vi "areaModify.vi"(3 "区域信息":T1 {"电极排列方式" items=["等间隔十字排列", "等间隔一字排列", "等间隔错误排列"]}, 8 "error in (no error)":errorcluster caption="错误输入（无错误）", 11 "编号":dbl) -> (0 "error out (no error) 2":errorcluster caption="错误输出（无错误）", 1 "连接的字符串":string)   [LabVIEW 2014, in "SettingD.lvlib"]
uses:
  SettingD.llb/SettingD.lvlib
  DataBase/DataBase.lvlib
panel:
  out "area_id":string
  out "结果字符串":string
  in  "取消按钮":bool
  in  "确定按钮":bool
  out "元素":string
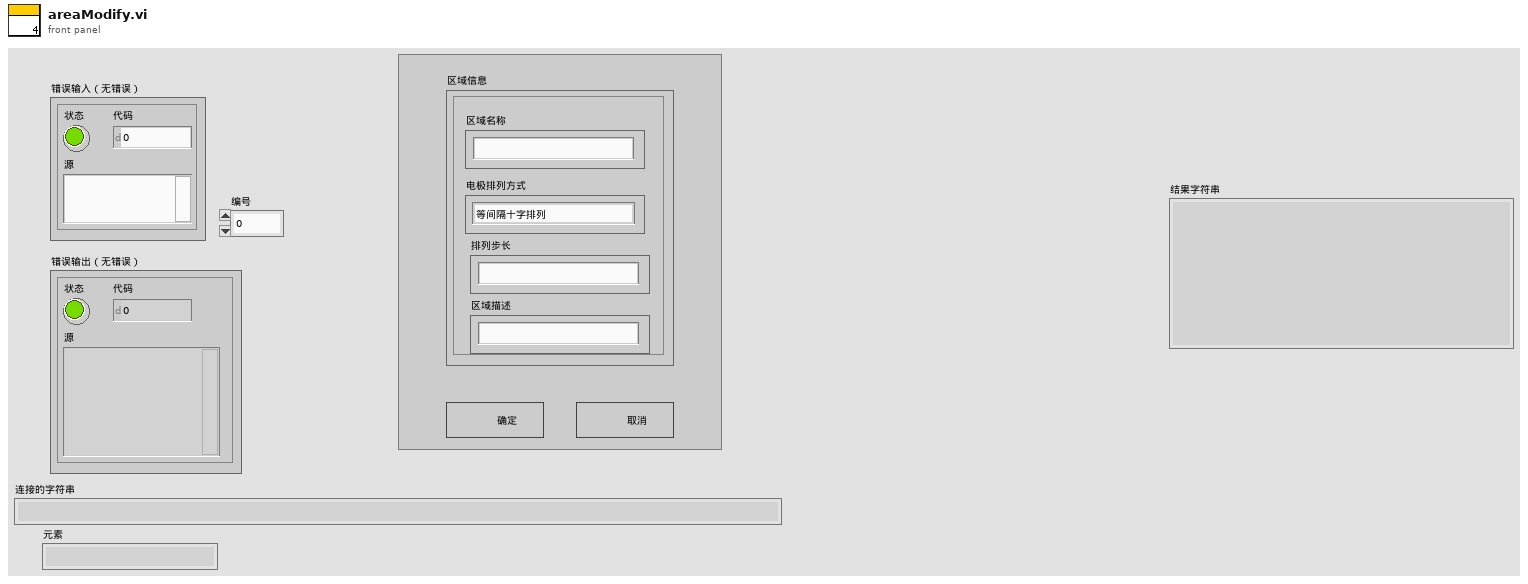
[diagram p1: front panel]
types:
  T1 = cluster{"区域名称":string, "电极排列方式":u16, "排列步长":string, "区域描述":string}
  T2 = cluster{"data":string, i32, "data":string, "data":string}
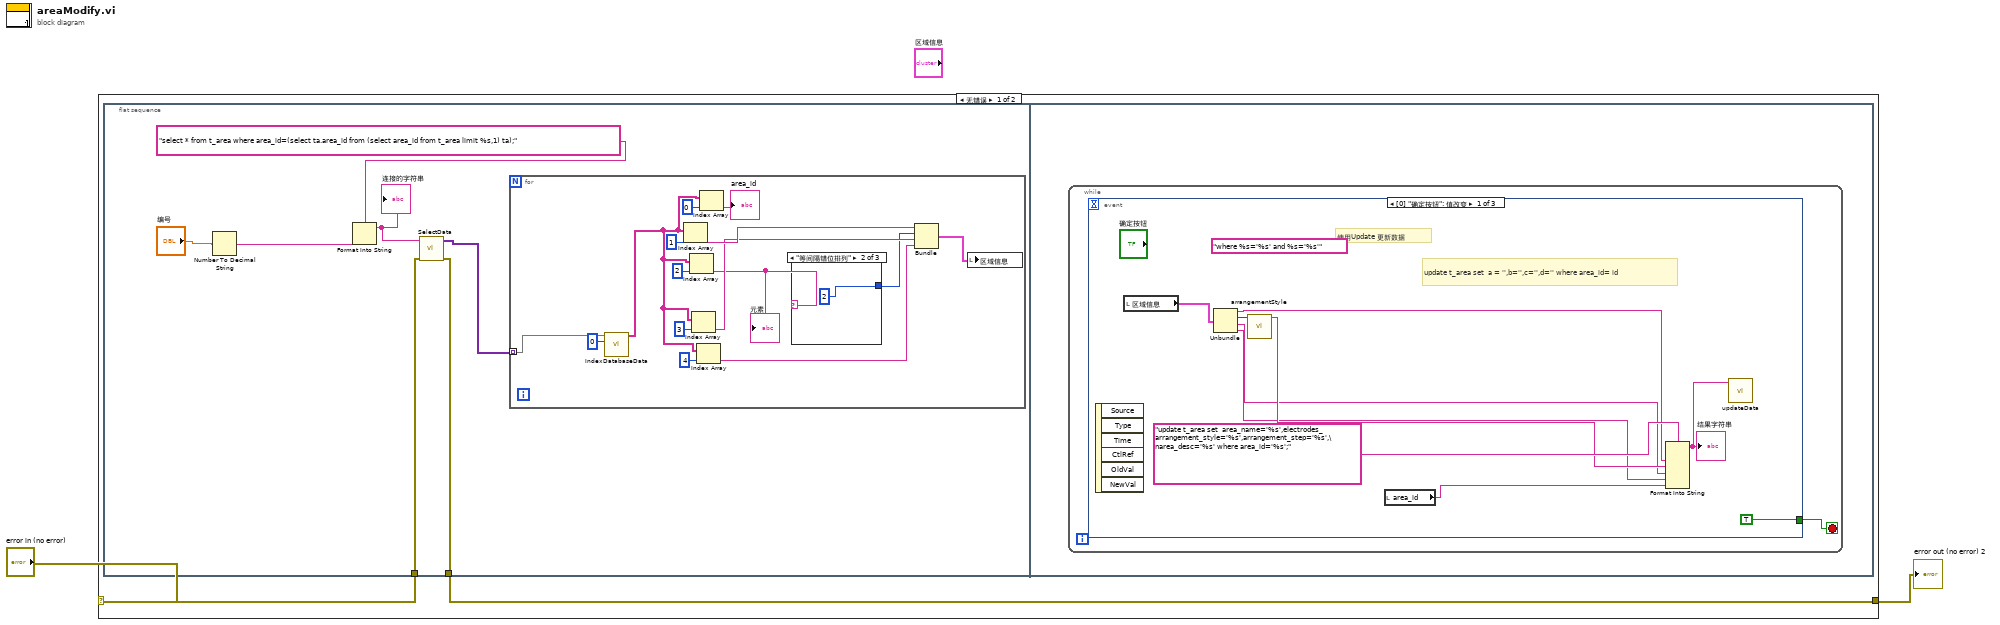
[diagram p0: block diagram]
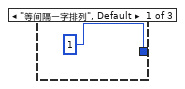
[diagram p2: hidden frame]
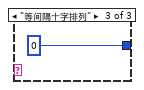
[diagram p3: hidden frame]
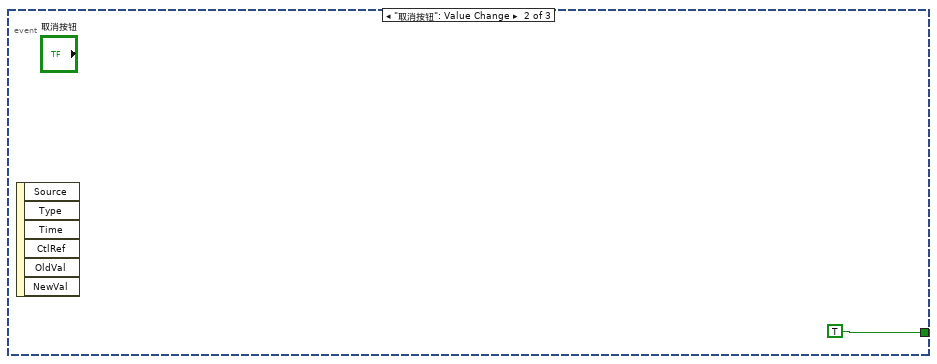
[diagram p4: hidden frame]
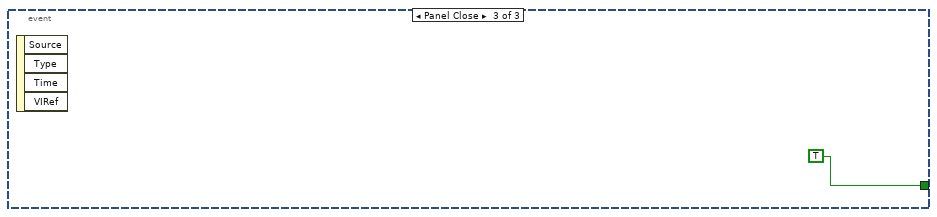
[diagram p5: hidden frame]
diagram:
  n1 = case shown="无错误" "error in (no error)" {
    selector: "error in (no error)" -> [w4 w43]
    tunnel: [w3 w43] -> w1
    frame No Error {
      n2 = flat-sequence {
        tunnel: w4 -> [w11]
        tunnel: [w10] -> w3
        frame #0 {
          n3 = Number To Decimal String(number="编号") -> (decimal integer string=w7:string)  [unwired: 1 in]
          n4 = Format Into String(format string="select * from t_area where area_id=(select ta.area_id from (select area_id from t_area limit %s,1) ta);" ("SQL query"), w7) -> (resulting string=w5:string)  [unwired: 2 in, 1 out]
          "连接的字符串" <- w5
          n5 = call "SelectData.vi"("SQL query"=w5, "error in"=w11) -> ("recordset data"=w9:variant[][], "error out"=w10:errorcluster)  [unwired: 6 in]
          n6 = for {
            tunnel: w9 -> [w26] mode=indexing
            n7 = call "IndexDatabaseData.vi"("index"=0, "recordset data"=w26) -> ("数组"=w15:string[])  [unwired: 9 in]
            n8 = Index Array(array=w15, index=1 ("索引")) -> (element=w21:string)
            n9 = Index Array(array=w15, index=2 ("索引")) -> (element=w18:string)
            "元素" <- w18
            n10 = Index Array(array=w15, index=3 ("索引")) -> (element=w20:string)
            n11 = Index Array(array=w15, index=4 ("索引")) -> (element=w19:string)
            n12 = Index Array(array=w15, index=0 ("索引")) -> (element=→"area_id":string)
            n13 = case shown="\"等间隔错位排列\"" w18 {
              tunnel: [1 2 0] -> w17
              frame "等间隔一字排列", Default {
              }
              frame "等间隔错位排列" {
              }
              frame "等间隔十字排列" {
              }
            }
            n14 = Bundle("data"=w21, w17, "data"=w20, "data"=w19) -> (w16:T2)  [unwired: 1 in]
            n15 = local write "区域信息"(w16) -> ()
          }
        }
        frame #1 {
          n16 = while {
            stop <- w30 stop-if-true
            n17 = event shown="[0] \"确定按钮\": 值改变" {
              selector: _ -> [_ _ _]
              dyn-events: _ -> [_ _ _]
              timeout: _ -> [_ _ _]
              tunnel: [TRUE TRUE TRUE] -> w30
              event "确定按钮": Value Change {
                (unwired) "where %s='%s' and %s='%s'" ("format string")
                # "update t_area set  a = '',b='',c='',d='' where area_id= id"
                # "使用Update 更新数据"
                n18 = event-data() -> ()  [unwired: 1 in, 6 out]
                n19 = local read "区域信息"() -> (w39:T1)
                n20 = Unbundle(w39) -> ("区域名称"=w36:string, "电极排列方式"=w38:u16, "排列步长"=w34:string, "区域描述"=w33:string)
                n21 = call "arrangementStyle.vi"("索引"=w38) -> ("排列方式"=w35:string)  [unwired: 10 in]
                n22 = local read "area_id"() -> (w31:string)
                n23 = Format Into String(format string="update t_area set  area_name='%s',electrodes_arrangement_style='%s',arrangement_step='%s',\narea_desc='%s' where area_id='%s';", w36, w35, w34, w33, w31) -> (resulting string=w32:string)  [unwired: 2 in, 1 out]
                "结果字符串" <- w32
                n24 = call "updateData.vi"("SQL query"=w32) -> ()  [unwired: 10 in, 1 out]
              }
              event "取消按钮": Value Change {
                n25 = event-data() -> ()  [unwired: 1 in, 6 out]
              }
              event Panel Close {
                n26 = event-data() -> ()  [unwired: 1 in, 4 out]
              }
            }
          }
        }
      }
    }
    frame Error {
    }
  }
  "error out (no error) 2" <- w1
